vi "ReadMeasurementFile.vi"(1 "Defragment (T)":bool=TRUE, 2 "MeasurementParameters.PXDConfig":T1[](array[typedef]), 6 "WritingOptions":T5=enum."High&Low32bit", 8 "error in (no error)":errorcluster, 11 "Path":path) -> (0 "error out":errorcluster, 5 "Threshold High Range 2":dbl[](array[numeric]), 7 "Threshold Low Range 2":dbl[](array[numeric]), 9 "ThrScan_RICE_High":u32[][](graph), 10 "ThrScan_RICE_Low":u16[][](graph))   [LabVIEW 2022 SP3]
uses:
  #typedef_PXD_FileWritingOption.ctl
  #typedef_PXDConfig.ctl
  #typedef_PixelParameters.ctl
  #typedef_PXD_DACs_Values.ctl
  #typedef_PXD_DACs_NumericValues.ctl
panel:
  out "transposed array":u16[][](array[numeric])
  out "size(s) 4":i32
  out "size(s) 3":i32
  out "size(s) 2":i32[](array[numeric])
  out "size(s)":i32[](array[numeric])
  out "x-y":u32
  in  "Threshold Low Range":dbl[](array[numeric])
  in  "Threshold High Range":dbl[](array[numeric])
  in  "ThresholdLow":u16[][](array[numeric])
  in  "ThresholdHigh":u32[][](array[numeric])
  # "0 - low gain, 1 - high gain"
  # "0 - OFF, 1 - ON"
  # "0 - OFF, 1 - ON"
  # "0- highest.  31 - lowest gain"
  # "0 - connected, 1 - disconnected"
  # "0- OFF, 1 - ON"
  # "0 - low gain, 1 - high gain"
  # "0 - low current, 1 - high current"
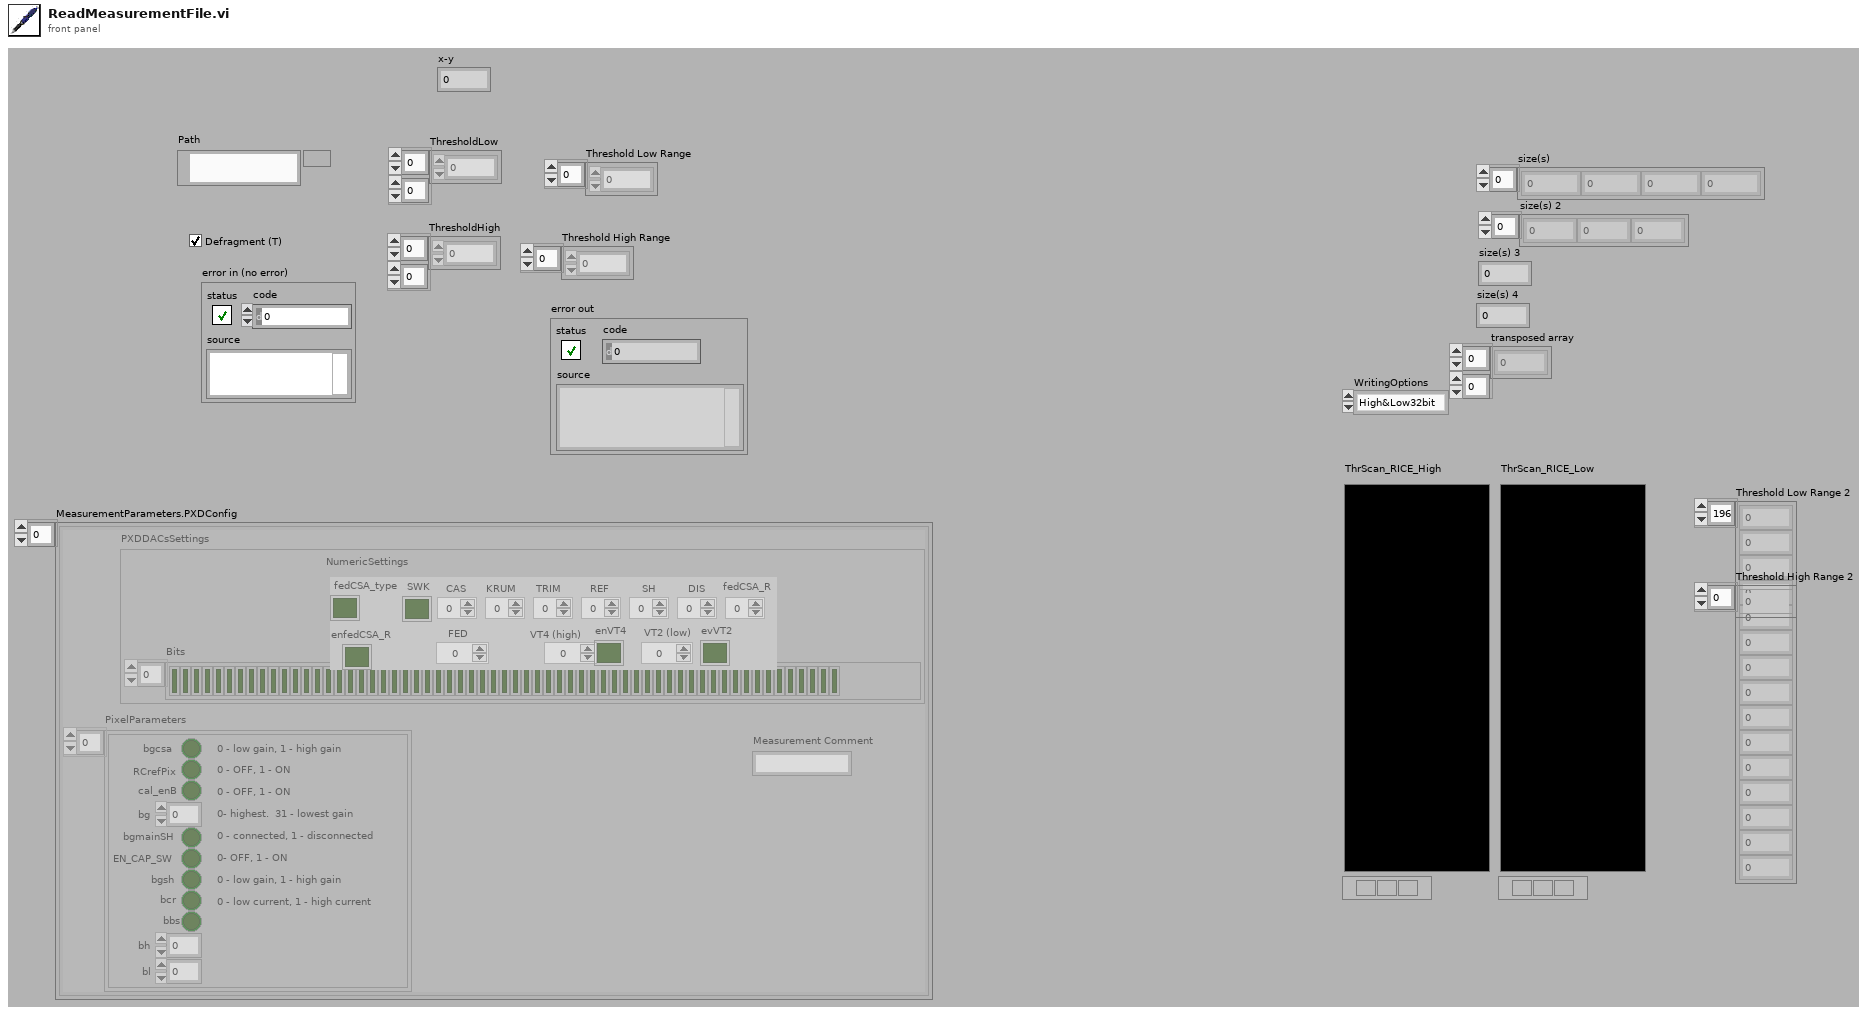
[diagram p1: front panel]
types:
  T1 = typedef "#typedef_PXDConfig.ctl" = cluster{"PixelParameters":T2[], "PXDDACsSettings":T3, "Measurement Comment":string}
  T2 = typedef "#typedef_PixelParameters.ctl" = cluster{"cal_enB":bool, "bg":u8, "bl":u8, "bcr":bool, "bbs":bool, "bh":u8, "bgcsa":bool, "EN_CAP_SW":bool, "bgsh":bool, "RCrefPix":bool, "bgmainSH":bool}
  T3 = typedef "#typedef_PXD_DACs_Values.ctl" = cluster{"Bits":bool[], "NumericSettings":T4}
  T4 = typedef "#typedef_PXD_DACs_NumericValues.ctl" = cluster{"fedCSA_type":bool, "CAS":i32, "KRUM":i32, "TRIM":i32, "REF":i32, "SH":i32, "DIS":i32, "fedCSA_R":i32, "enfedCSA_R":bool, "FED":i32, "VT4 (high)":i32, "enVT4":bool, "VT2 (low)":i32, "evVT2":bool, "SWK":bool}
  T5 = typedef "#typedef_PXD_FileWritingOption.ctl" = enum16{"OnlyLow32bit", "OnlyLow16bit", "OnlyHigh16bit", "High&Low16bit", "High&Low32bit"}
  T6 = enum16{"open", "open or create", "create or replace", "create", "open (read-only)"}
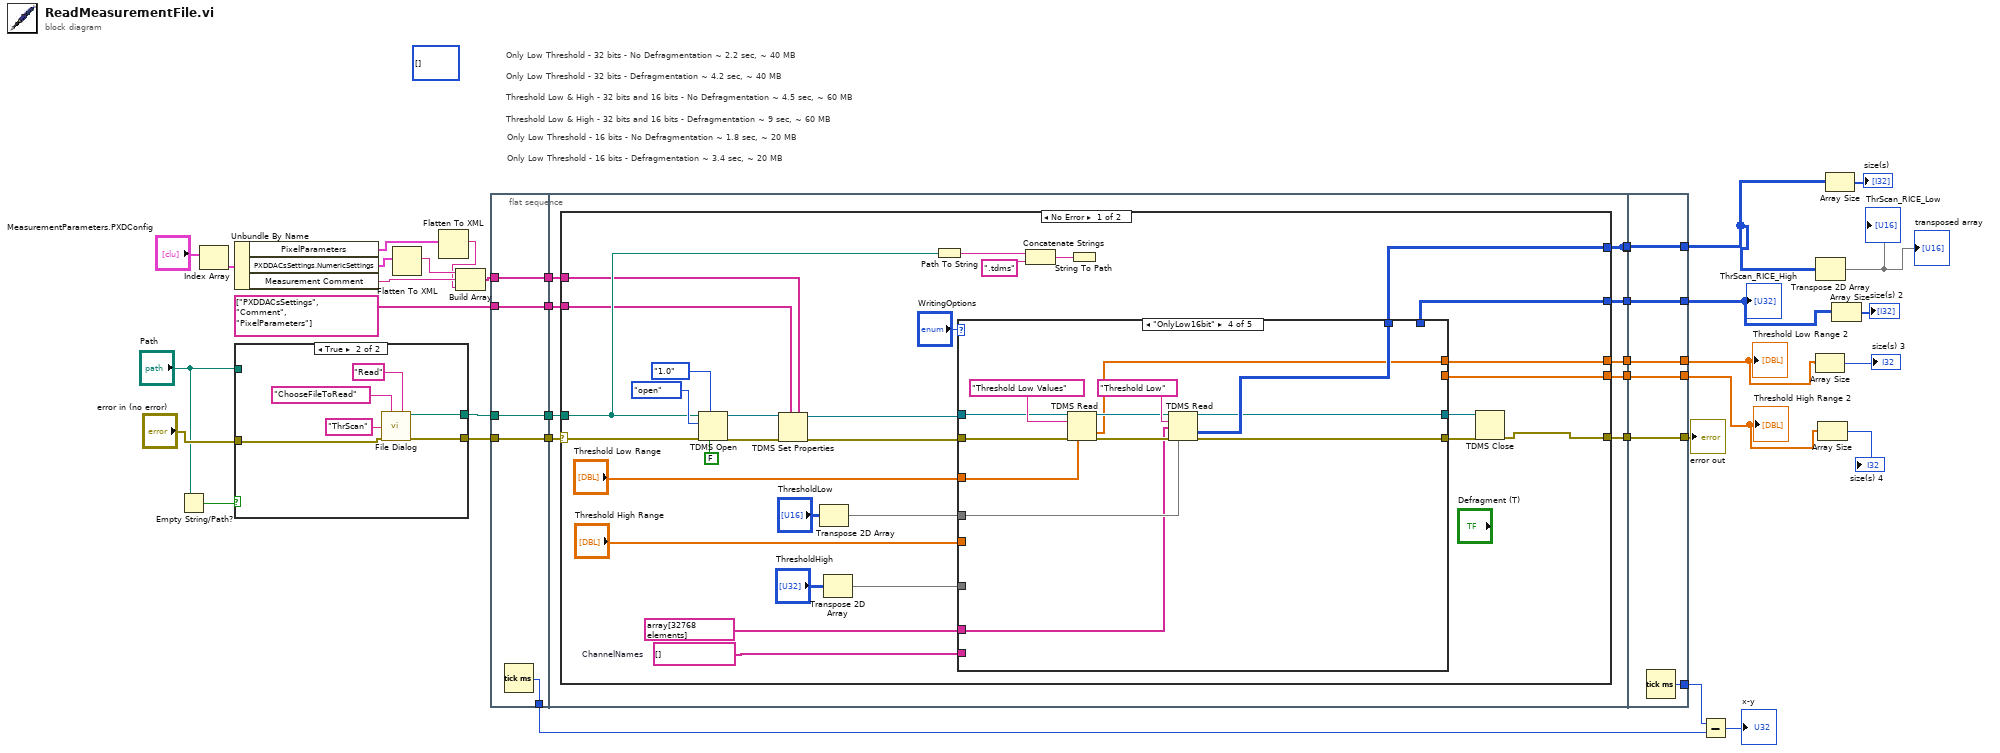
[diagram p0: block diagram]
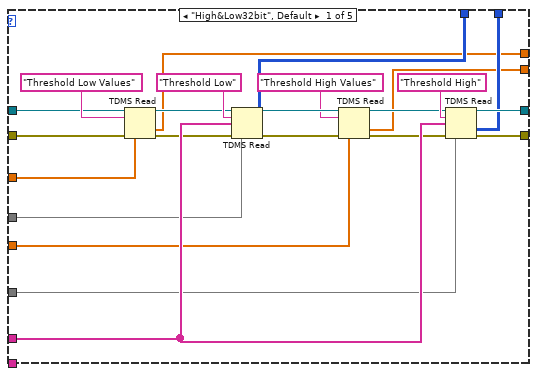
[diagram p2: hidden frame]
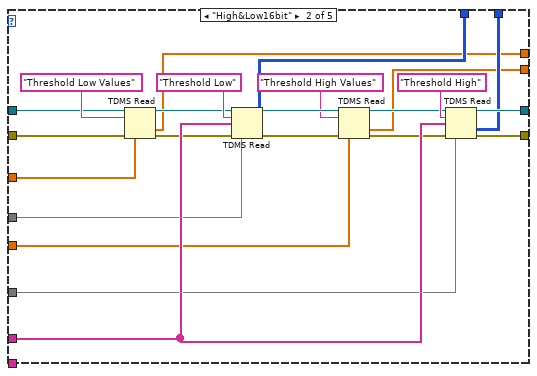
[diagram p3: hidden frame]
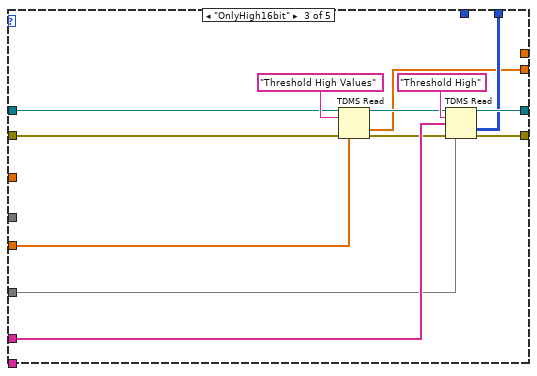
[diagram p4: hidden frame]
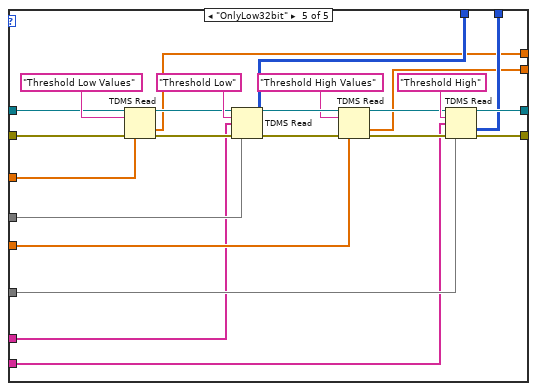
[diagram p5: hidden frame]
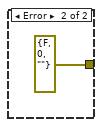
[diagram p6: hidden frame]
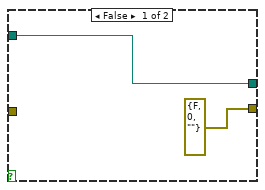
[diagram p7: hidden frame]
diagram:
  (unwired) u16[][] []
  # "Only Low Threshold - 16 bits - Defragmentation ~ 3.4 sec, ~ 20 MB"
  # "Only Low Threshold - 16 bits - No Defragmentation ~ 1.8 sec, ~ 20 MB"
  # "Threshold Low & High - 32 bits and 16 bits - Defragmentation ~ 9 sec, ~ 60 MB"
  # "Threshold Low & High - 32 bits and 16 bits - No Defragmentation ~ 4.5 sec, ~ 60 MB"
  # "Only Low Threshold - 32 bits - Defragmentation ~ 4.2 sec, ~ 40 MB"
  # "Only Low Threshold - 32 bits - No Defragmentation ~ 2.2 sec, ~ 40 MB"
  n1 = Empty String/Path?(string/path="Path") -> (empty?=w4:bool)
  n2 = Index Array(array="MeasurementParameters.PXDConfig") -> (element=w26:T1)  [unwired: 1 in]
  n3 = Unbundle By Name(w26) -> ("PixelParameters"=w18:T2[], "PXDDACsSettings.NumericSettings"=w20:T4, "Measurement Comment"=w21:string)
  n4 = case shown="True" w4 {
    tunnel: "Path" -> [w39 _]
    tunnel: [errorcluster {"status"=FALSE, "code"=0, "source"=""} ("error out") w42] -> w34
    tunnel: [w39 w41] -> w35
    tunnel: "error in (no error)" -> [_ w40]
    frame False {
    }
    frame True {
      n5 = call "File Dialog"("prompt"="ChooseFileToRead", "button label"="Read", "default name"="ThrScan", "error in"=w40) -> ("selected path"=w41:path, "error out"=w42:errorcluster)  [unwired: 3 in, 7 out]
    }
  }
  n6 = Flatten To XML(6:w20) -> (2:w19:string)
  n7 = Flatten To XML(6:w18) -> (2:w17:string)
  n8 = Build Array(w19, w21, w17) -> (w24:string[])
  n9 = flat-sequence {
    tunnel: w34 -> [w49]
    tunnel: w35 -> [w50]
    tunnel: [w50] -> w32
    tunnel: [w49] -> w31
    tunnel: [w48] -> w29
    tunnel: [w47] -> w25
    tunnel: w24 -> [w47]
    tunnel: string[] ["PXDDACsSettings", "Comment", "PixelParameters"] ("property names") -> [w46]
    tunnel: [w46] -> w23
    tunnel: [w59] -> w33
    tunnel: w32 -> [w58]
    tunnel: w31 -> [w57]
    tunnel: w25 -> [w56]
    tunnel: w23 -> [w55]
    tunnel: [w54] -> w16
    tunnel: [w53] -> w15
    tunnel: [w53] -> w14
    tunnel: [w52] -> w13
    tunnel: [w51] -> w12
    tunnel: [w192] -> w37
    tunnel: w33 -> [w192]
    tunnel: [w191] -> w30
    tunnel: w16 -> [w190]
    tunnel: [w190] -> w3
    tunnel: [w189] -> w2
    tunnel: w15 -> [_]
    tunnel: w14 -> [w189]
    tunnel: [w188] -> w8
    tunnel: w13 -> [w188]
    tunnel: w12 -> [w187]
    tunnel: [w187] -> w9
    frame #0 {
      n10 = Tick Count (ms)() -> (millisecond timer value=w48:u32)
    }
    frame #1 {
      n11 = case shown="No Error" w57 {
        selector: w57 -> [w77 _]
        tunnel: [w60 errorcluster {"status"=FALSE, "code"=0, "source"=""} ("error out")] -> w59
        tunnel: w58 -> [w78 _]
        tunnel: w56 -> [w69 _]
        tunnel: w55 -> [w68 _]
        tunnel: [w64 _] -> w54
        tunnel: [w63 _] -> w53
        tunnel: [w62 _] -> w52
        tunnel: [w61 _] -> w51
        frame No Error {
          w76 = string[] []  # ChannelNames
          n12 = TDMS Open(6:FALSE ("disable buffering (T)"), 7:enum16{"1.0", "2.0"}."1.0" ("file format version (2.0)"), 8:w77, 10:T6."open" ("operation (0:open)"), 11:w78) -> (0:w70:errorcluster, 3:w71:refnum<k34>)  [unwired: 2 in]
          n13 = TDMS Set Properties(5:w69, 7:w68, 8:w70, 11:w71) -> (0:w66:errorcluster, 3:w67:refnum<k34>)  [unwired: 2 in, 2 out]
          n14 = Transpose 2D Array(2D array="ThresholdLow") -> (transposed array=w75:u16[][])
          n15 = Transpose 2D Array(2D array="ThresholdHigh") -> (transposed array=w74:u32[][])
          n16 = Path To String(path=w78) -> (string=w87:string)
          n17 = case shown="\"OnlyLow16bit\"" "WritingOptions" {
            tunnel: w74 -> [w94 w117 w140 _ w169]
            tunnel: w75 -> [w96 w119 _ w155 w171]
            tunnel: w67 -> [w101 w124 w137 w158 w175]
            tunnel: w66 -> [w100 w123 w136 w157 w174]
            tunnel: [w110 w133 w147 w149 w183] -> w82
            tunnel: [w103 w126 w144 w150 w176] -> w81
            tunnel: "Threshold High Range" -> [w95 w118 w141 _ w170]
            tunnel: "Threshold Low Range" -> [w97 w120 _ w152 w164]
            tunnel: string[] array[32768 elements] ("Array") -> [w102 w125 w143 w151 w162]
            tunnel: w76 -> [_ _ _ _ w163]
            tunnel: [w93 w116 w139 _ w168] -> w64
            tunnel: [w92 w115 _ w154 w167] -> w63
            tunnel: [w91 w114 _ w153 w166] -> w62
            tunnel: [w90 w113 w138 _ w165] -> w61
            frame "High&Low32bit", Default {
              n18 = TDMS Read(0:w101, 5:"Threshold Low Values" ("group name in (Untitled)"), 11:w100, 12:w97) -> (4:w109:refnum<k34>, 10:w91:dbl[], 15:w99:errorcluster)  [unwired: 4 in, 3 out]
              n19 = TDMS Read(0:w109, 5:"Threshold Low" ("group name in (Untitled)"), 7:w102, 11:w99, 12:w96) -> (4:w108:refnum<k34>, 10:w92:u16[][], 15:w106:errorcluster)  [unwired: 3 in, 3 out]
              n20 = TDMS Read(0:w108, 5:"Threshold High Values" ("group name in (Untitled)"), 11:w106, 12:w95) -> (4:w107:refnum<k34>, 10:w90:dbl[], 15:w98:errorcluster)  [unwired: 4 in, 3 out]
              n21 = TDMS Read(0:w107, 5:"Threshold High" ("group name in (Untitled)"), 7:w102, 11:w98, 12:w94) -> (4:w110:refnum<k34>, 10:w93:u32[][], 15:w103:errorcluster)  [unwired: 3 in, 3 out]
            }
            frame "High&Low16bit" {
              n22 = TDMS Read(0:w124, 5:"Threshold Low Values" ("group name in (Untitled)"), 11:w123, 12:w120) -> (4:w132:refnum<k34>, 10:w114:dbl[], 15:w122:errorcluster)  [unwired: 4 in, 3 out]
              n23 = TDMS Read(0:w132, 5:"Threshold Low" ("group name in (Untitled)"), 7:w125, 11:w122, 12:w119) -> (4:w131:refnum<k34>, 10:w115:u16[][], 15:w129:errorcluster)  [unwired: 3 in, 3 out]
              n24 = TDMS Read(0:w131, 5:"Threshold High Values" ("group name in (Untitled)"), 11:w129, 12:w118) -> (4:w130:refnum<k34>, 10:w113:dbl[], 15:w121:errorcluster)  [unwired: 4 in, 3 out]
              n25 = TDMS Read(0:w130, 5:"Threshold High" ("group name in (Untitled)"), 7:w125, 11:w121, 12:w117) -> (4:w133:refnum<k34>, 10:w116:u32[][], 15:w126:errorcluster)  [unwired: 3 in, 3 out]
            }
            frame "OnlyHigh16bit" {
              n26 = TDMS Read(0:w137, 5:"Threshold High Values" ("group name in (Untitled)"), 11:w136, 12:w141) -> (4:w146:refnum<k34>, 10:w138:dbl[], 15:w142:errorcluster)  [unwired: 4 in, 3 out]
              n27 = TDMS Read(0:w146, 5:"Threshold High" ("group name in (Untitled)"), 7:w143, 11:w142, 12:w140) -> (4:w147:refnum<k34>, 10:w139:u32[][], 15:w144:errorcluster)  [unwired: 3 in, 3 out]
            }
            frame "OnlyLow16bit" {
              n28 = TDMS Read(0:w158, 5:"Threshold Low Values" ("group name in (Untitled)"), 11:w157, 12:w152) -> (4:w160:refnum<k34>, 10:w153:dbl[], 15:w156:errorcluster)  [unwired: 4 in, 3 out]
              n29 = TDMS Read(0:w160, 5:"Threshold Low" ("group name in (Untitled)"), 7:w151, 11:w156, 12:w155) -> (4:w149:refnum<k34>, 10:w154:u16[][], 15:w150:errorcluster)  [unwired: 3 in, 3 out]
            }
            frame "OnlyLow32bit" {
              n30 = TDMS Read(0:w175, 5:"Threshold Low Values" ("group name in (Untitled)"), 11:w174, 12:w164) -> (4:w182:refnum<k34>, 10:w166:dbl[], 15:w173:errorcluster)  [unwired: 4 in, 3 out]
              n31 = TDMS Read(0:w182, 5:"Threshold Low" ("group name in (Untitled)"), 7:w162, 11:w173, 12:w171) -> (4:w181:refnum<k34>, 10:w167:u16[][], 15:w179:errorcluster)  [unwired: 3 in, 3 out]
              n32 = TDMS Read(0:w181, 5:"Threshold High Values" ("group name in (Untitled)"), 11:w179, 12:w170) -> (4:w180:refnum<k34>, 10:w165:dbl[], 15:w172:errorcluster)  [unwired: 4 in, 3 out]
              n33 = TDMS Read(0:w180, 5:"Threshold High" ("group name in (Untitled)"), 7:w163, 11:w172, 12:w169) -> (4:w183:refnum<k34>, 10:w168:u32[][], 15:w176:errorcluster)  [unwired: 3 in, 3 out]
            }
          }
          n34 = Concatenate Strings(w87, ".tdms" ("string")) -> (w88:string)
          n35 = String To Path(string=w88) -> ()  [unwired: 1 out]
          n36 = TDMS Close(8:w81, 11:w82) -> (0:w60:errorcluster)  [unwired: 1 out]
        }
        frame Error {
        }
      }
    }
    frame #2 {
      n37 = Tick Count (ms)() -> (millisecond timer value=w191:u32)
    }
  }
  n38 = Subtract(x=w30, y=w29) -> (x-y=→"x-y":u32)
  n39 = Array Size(array=w8) -> (size(s)=→"size(s) 3":i32)
  n40 = Transpose 2D Array(2D array=w2) -> (transposed array=→"ThrScan_RICE_Low" →"transposed array":u16[][])
  n41 = Array Size(array=w9) -> (size(s)=→"size(s) 4":i32)
  n42 = Array Size(array=w2) -> (size(s)=→"size(s)":i32[])
  n43 = Array Size(array=w3) -> (size(s)=→"size(s) 2":i32[])
  "error out" <- w37
  "ThrScan_RICE_High" <- w3
  "Threshold High Range 2" <- w9
  "Threshold Low Range 2" <- w8
